vi "StopSignal-TestMain.vi"() -> ()   [LabVIEW 2017, in "StopSignal.lvlib"]
uses:
  StopSignal.lvlib
panel:
  out "reason #4":string
  out "reason #1":string
  out "reason #2":string
  out "reason #3":string
  out "current time":timestamp
  in  "stop":bool
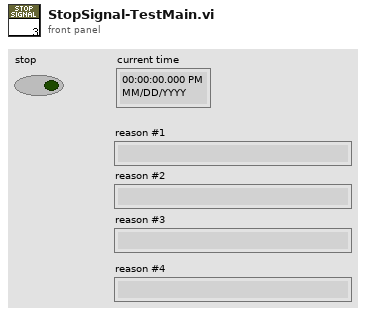
[diagram p1: front panel]
types:
  T1 = typedef "StopSignal.lvlib/StopSignal.ctl" = refnum<k1>
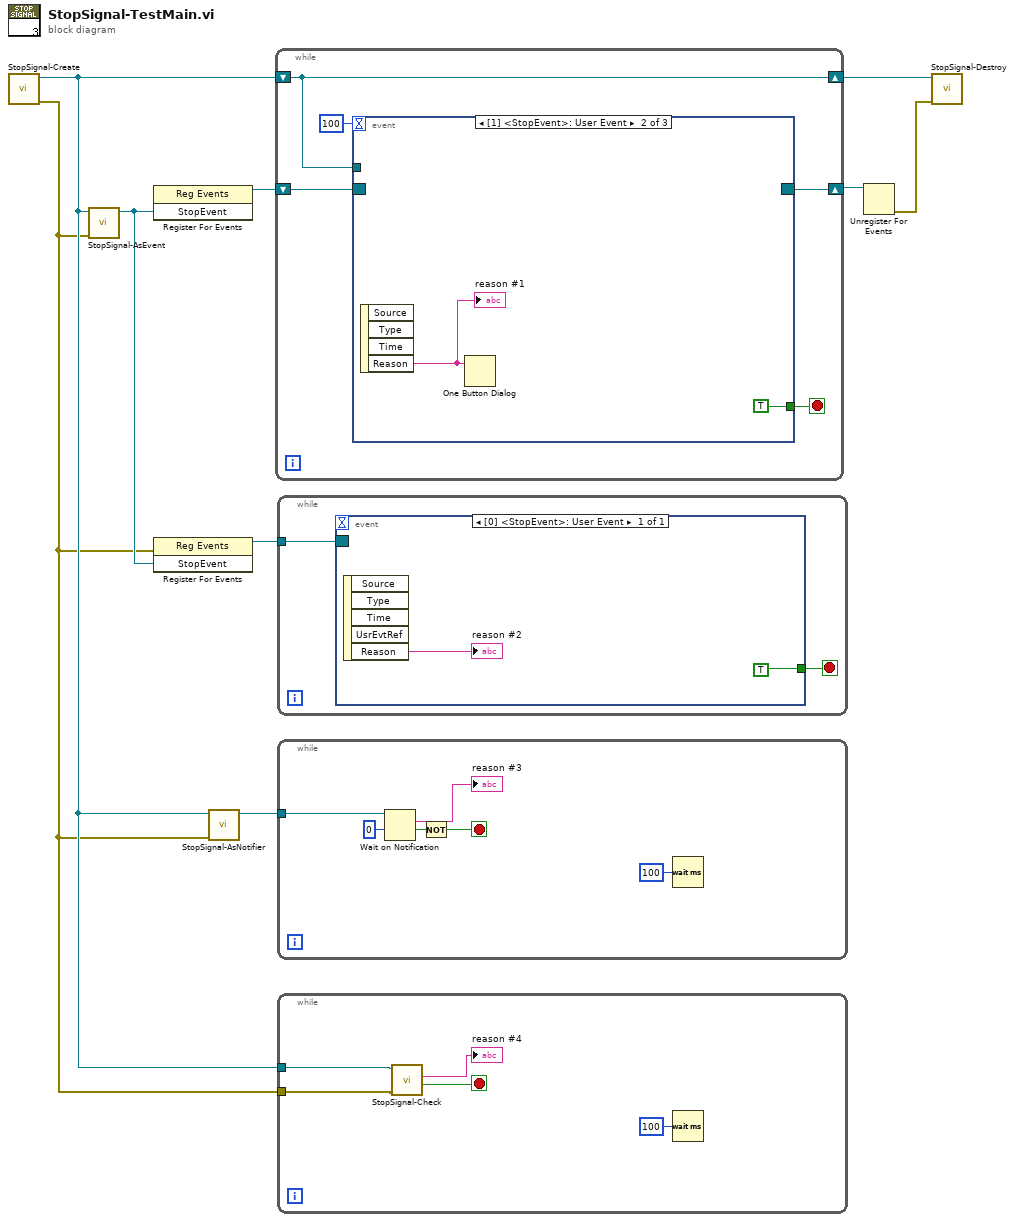
[diagram p0: block diagram]
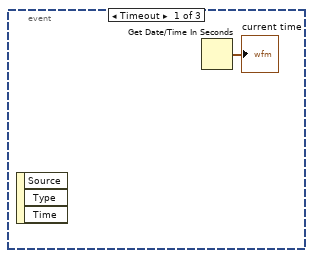
[diagram p2: hidden frame]
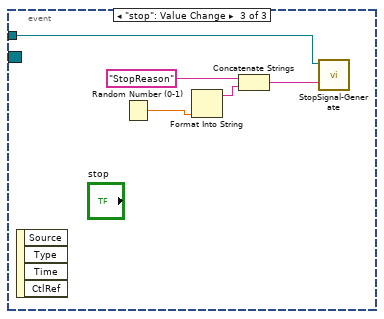
[diagram p3: hidden frame]
diagram:
  n1 = call "StopSignal-Create.vi"() -> ("error out"=w1:errorcluster, "StopSignal"=w2:T1)  [unwired: 10 in]
  n2 = call "StopSignal-AsEvent.vi"("error in (no error)"=w1, "StopSignal"=w2) -> ("StopEvent"=w5:refnum<user-event>)  [unwired: 8 in, 1 out]
  n3 = register-events(w5) -> (reference out=w9:refnum<event-registration>)  [unwired: 2 in, 1 out]
  n4 = register-events(error in=w1, w5) -> (reference out=w7:refnum<event-registration>)  [unwired: 1 in, 1 out]
  n5 = call "StopSignal-AsNotifier.vi"("error in (no error)"=w1, "StopSignal"=w2) -> ("StopNotifier"=w3:refnum<notifier>)  [unwired: 8 in, 1 out]
  n6 = while {
    shift-right: [w11] -> w8
    shift-left: w9 -> [w14]
    shift-right: [w10] -> w4
    shift-left: w2 -> [w10]
    stop <- w13 stop-if-true
    n7 = event shown="[1] <StopEvent>: User Event" {
      selector: w14 -> [_ _ _]
      dyn-events: [_ _ _] -> w11
      timeout: 100 -> [_ _ _]
      tunnel: [_ TRUE _] -> w13
      tunnel: w10 -> [_ _ w18]
      event Timeout {
        n8 = event-data() -> ()  [unwired: 1 in, 3 out]
        n9 = Get Date/Time In Seconds() -> (seconds since 1Jan1904=→"current time":timestamp)
      }
      event User Event {
        n10 = event-data() -> ("Reason"=w16:string)  [unwired: 1 in, 3 out]
        "reason #1" <- w16
        n11 = One Button Dialog(message=w16) -> ()  [unwired: 1 in, 1 out]
      }
      event "stop": Value Change {
        n12 = event-data() -> ()  [unwired: 1 in, 4 out]
        n13 = Random Number (0-1)() -> (number: 0 to 1=w21:dbl)
        n14 = Format Into String(w21) -> (resulting string=w20:string)  [unwired: 3 in, 1 out]
        n15 = Concatenate Strings("StopReason" ("event data"), w20) -> (w19:string)
        n16 = call "StopSignal-Generate.vi"("reason(\"\")"=w19, "StopSignal"=w18) -> ()  [unwired: 8 in, 2 out]
      }
    }
  }
  n17 = while {
    tunnel: w7 -> [w24]
    stop <- w23 stop-if-true
    n18 = event shown="[0] <StopEvent>: User Event" {
      selector: w24 -> [_]
      dyn-events: _ -> [_]
      timeout: _ -> [_]
      tunnel: [TRUE] -> w23
      event User Event {
        n19 = event-data() -> ("Reason"=→"reason #2":string)  [unwired: 1 in, 4 out]
      }
    }
  }
  n20 = while {
    tunnel: w3 -> [w27]
    stop <- w28 stop-if-true
    n21 = Wait on Notification(notifier=w27, timeout in ms (-1)=0) -> (notification=→"reason #3":string, timed out?=w31:bool)  [unwired: 2 in, 2 out]
    n22 = Not(x=w31) -> (.not. x?=w28:bool)
    n23 = Wait (ms)(milliseconds to wait=u32 100) -> ()  [unwired: 1 out]
  }
  n24 = while {
    tunnel: w2 -> [w36]
    tunnel: w1 -> [w35]
    stop <- w34 stop-if-true
    n25 = call "StopSignal-Check.vi"("error in (no error)"=w35, "StopSignal"=w36) -> ("Stop?"=w34:bool, "Reason"=→"reason #4":string)  [unwired: 6 in, 2 out]
    n26 = Wait (ms)(milliseconds to wait=u32 100) -> ()  [unwired: 1 out]
  }
  n27 = Unregister For Events(event registration refnum=w8) -> (error out=w6:errorcluster)  [unwired: 1 in]
  n28 = call "StopSignal-Destroy.vi"("error in (no error)"=w6, "StopSignal"=w4) -> ()  [unwired: 9 in, 1 out]
